vi "AV Write Single.vi"(8 "error in":errorcluster, 9 "Channel Index":i32=1, 10 "Flow AV":dbl, 11 "Flow Actual Value in":refnum<class "Flow Actual Value.lvclass">) -> (0 "error out":errorcluster, 3 "Flow Actual Value out":refnum<class "Flow Actual Value.lvclass">)   [LabVIEW 2023, in "Flow Actual Value.lvclass"]
uses:
  Flow Actual Value.lvclass
  Flow Actual Value.lvclass/Flow Actual Value.ctl
  Parents/Actual Value/Actual Value.lvclass
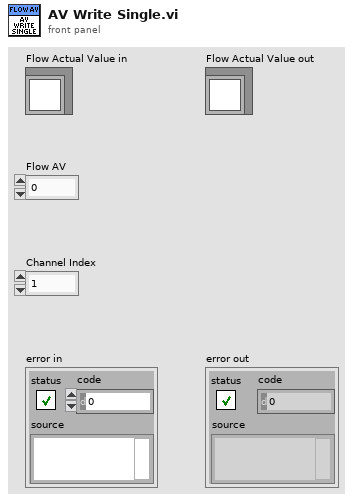
[diagram p1: front panel]
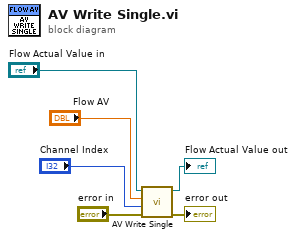
[diagram p0: block diagram]
diagram:
  n1 = call-parent "AV Write Single.vi"("error in"="error in", "Channel Index"="Channel Index", "Actual Value"="Flow AV", "Actual Value in"="Flow Actual Value in") -> ("error out"=→"error out":errorcluster, "Actual Value out"=→"Flow Actual Value out":refnum<class "Flow Actual Value.lvclass">)  [unwired: 6 in]
